vi "Set enable state.vi"(8 "Error in":errorcluster, 10 "Controls and indicators":T2, 11 "App state":T1) -> (0 "Error out":errorcluster, 3 "App state":T1)   [LabVIEW 2021]
uses:
  Typedefs/Control and indicators refs.ctl
  Typedefs/State.ctl
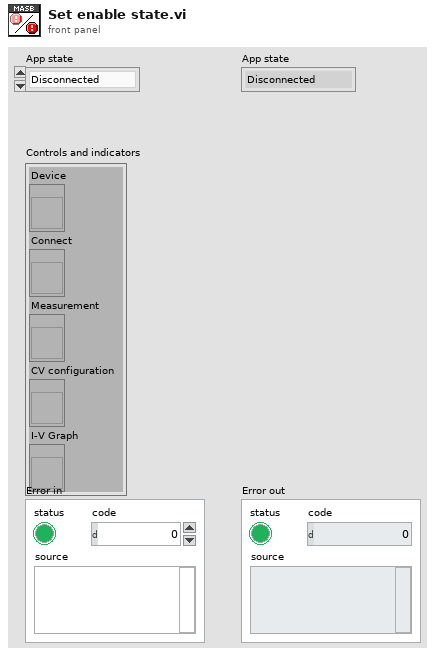
[diagram p1: front panel]
types:
  T1 = typedef "State.ctl" = enum16{"Disconnected", "Connected", "Measuring"}
  T2 = typedef "Control and indicators refs.ctl" = cluster{"Device":refnum<vi>, "Connect":refnum<vi>, "Measurement":refnum<vi>, "CV configuration":refnum<vi>, "I-V Graph":refnum<vi>}
  T3 = enum8{"Enabled", "Disabled", "Disabled and Grayed Out"}
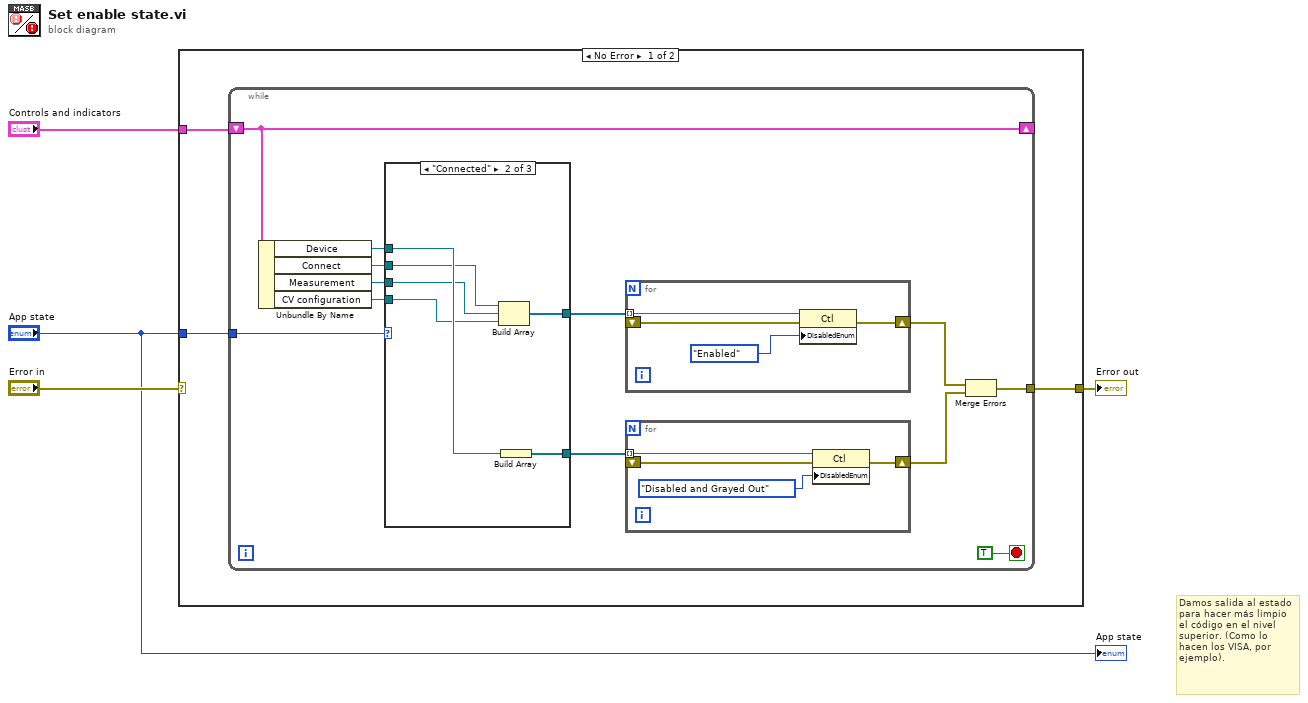
[diagram p0: block diagram]
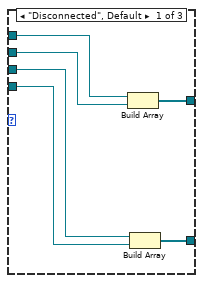
[diagram p2: hidden frame]
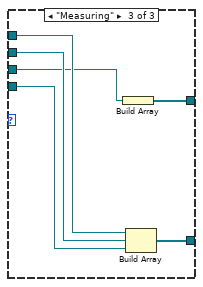
[diagram p3: hidden frame]
diagram:
  # "Damos salida al estado para hacer más limpio el código en el nivel superior. (Como lo hacen los VISA, por ejemplo)."
  n1 = case shown="No Error" "Error in" {
    selector: "Error in" -> [_ w46]
    tunnel: [w7 w46] -> w2
    tunnel: "App state" -> [w6 _]
    tunnel: "Controls and indicators" -> [w5 _]
    frame No Error {
      n2 = while {
        tunnel: [w19] -> w7
        shift-right: [w15] -> _
        shift-left: w5 -> [w15]
        tunnel: w6 -> [w16]
        stop <- TRUE stop-if-true
        n3 = Unbundle By Name(w15) -> ("Device"=w13:refnum<vi>, "Connect"=w12:refnum<vi>, "Measurement"=w11:refnum<vi>, "CV configuration"=w8:refnum<vi>)
        n4 = case shown="\"Connected\"" w16 {
          tunnel: [w33 w35 w42] -> w10
          tunnel: [w32 w39 w41] -> w9
          tunnel: w13 -> [w31 w38 w45]
          tunnel: w12 -> [w29 w37 w44]
          tunnel: w11 -> [w30 w36 w43]
          tunnel: w8 -> [w28 w34 w40]
          frame "Disconnected", Default {
            n5 = Build Array(w31, w29) -> (w33:refnum<vi>[])
            n6 = Build Array(w30, w28) -> (w32:refnum<vi>[])
          }
          frame "Connected" {
            n7 = Build Array(w37, w36, w34) -> (w35:refnum<vi>[])
            n8 = Build Array(w38) -> (w39:refnum<vi>[])
          }
          frame "Measuring" {
            n9 = Build Array(w43) -> (w42:refnum<vi>[])
            n10 = Build Array(w45, w44, w40) -> (w41:refnum<vi>[])
          }
        }
        n11 = for {
          shift-right: [w22] -> w14
          shift-left: _ -> [w23]
          tunnel: w10 -> [w20] mode=indexing
          n12 = property class="Ctl"(reference=w20, error in=w23, "DisabledEnum"=T3."Enabled" ("Disabled")) -> (error out=w22:errorcluster)  [unwired: 1 out]
        }
        n13 = for {
          shift-right: [w27] -> w18
          shift-left: _ -> [w26]
          tunnel: w9 -> [w24] mode=indexing
          n14 = property class="Ctl"(reference=w24, error in=w26, "DisabledEnum"=T3."Disabled and Grayed Out" ("Disabled")) -> (error out=w27:errorcluster)  [unwired: 1 out]
        }
        n15 = Merge Errors(w14, w18) -> (w19:errorcluster)
      }
    }
    frame Error {
    }
  }
  "Error out" <- w2
  "App state" <- "App state"
